vi "ini Ctrl_Str.vi"(7 "Select":enum16{"Save", "Load"}(ring), 8 "에러 입력":errorcluster caption="에러 입력(에러 없음)", 9 "값":string, 10 "키":string, 11 "섹션":string) -> (0 "에러 출력":errorcluster, 1 "값":string, 2 "경로 출력":path)   [LabVIEW 2020]
uses:
  Controls/Cmd_File path.ctl
  Controls/Cmd_File Type.ctl
  <vilib>/Utility/config.llb/Write Key (String).vi
  <vilib>/Utility/config.llb/Read Key (String).vi
  <vilib>/Utility/config.llb/NI_LVConfig.lvlib
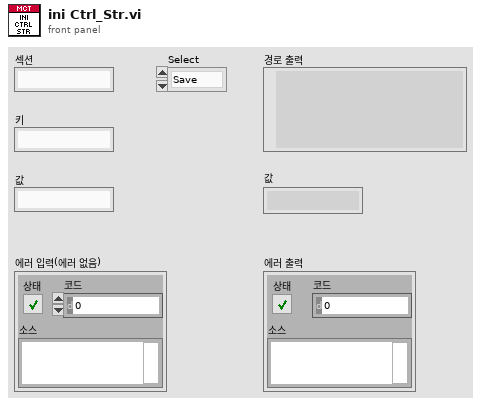
[diagram p1: front panel]
types:
  T1 = typedef "Cmd_File Type.ctl" = enum16{"엑셀", "엑셀(2003)", "텍스트", "설정", "2진", "VI", "CSV", "LOG", "폴더"}
  T2 = typedef "Cmd_File path.ctl" = enum16{"에러로그", "데이터파일경로", "성적서원본", "지난성적서", "Data Files", "경로생성", "Updater", "Template", "설정파일경로", "FTP Upload", "Update 경로", "어플리케이션"}
  T3 = typedef "NI_LVConfig.lvlib/Config Data RefNum.ctl" = refnum<k1>
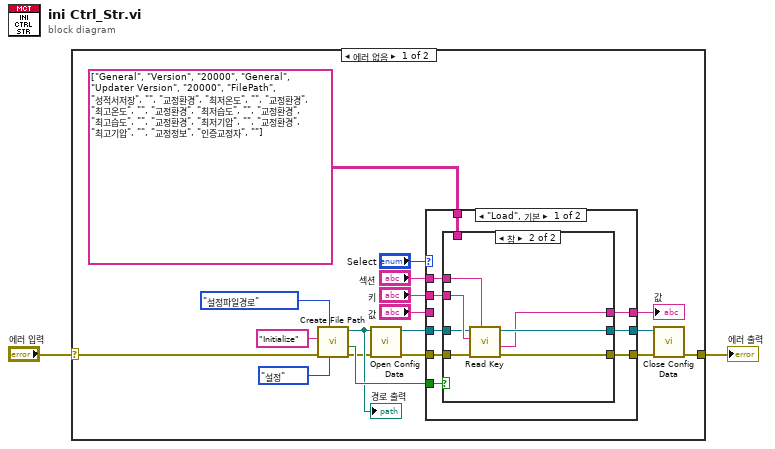
[diagram p0: block diagram]
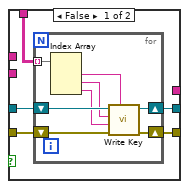
[diagram p2: hidden frame]
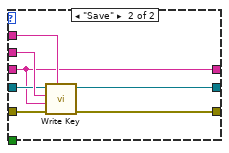
[diagram p3: hidden frame]
diagram:
  n1 = case shown="에러 없음" "에러 입력" {
    selector: "에러 입력" -> [w17 w57]
    tunnel: [w8 w57] -> w2
    frame No Error {
      n2 = call "Create File Path.vi"("파일타입"=Cmd_File_Type."설정", "항목"=Cmd_File_path."설정파일경로", "에러 입력"=w17, "문자열 in"="Initialize") -> ("error out"=w12:errorcluster, "파일존재?"=w15:bool, "파일경로"=w13:path)  [unwired: 4 in, 1 out]
      "경로 출력" <- w13
      n3 = call <vilib>:"Open Config Data.vi"("error in (no error)"=w12, "configuration file path"=w13) -> ("error out"=w10:errorcluster, "refnum"=w11:T3)  [unwired: 7 in, 1 out]
      n4 = case shown="\"Load\", 기본" "Select" {
        tunnel: [w27 w51] -> w9
        tunnel: "키" -> [w24 w56]
        tunnel: "섹션" -> [w25 w55]
        tunnel: w10 -> [w29 w54]
        tunnel: w11 -> [w28 w53]
        tunnel: w15 -> [w26 _]
        tunnel: string[][] [["General", "Version", "20000"], ["General", "Updater Version", "20000"], ["FilePath", "성적서저장", ""], ["교정환경", "최저온도", ""], ["교정환경", "최고온도", ""], ["교정환경", "최저습도", ""], ["교정환경", "최고습도", ""], ["교정환경", "최저기압", ""], ["교정환경", "최고기압", ""], ["교정정보", "인증교정자", ""]] -> [w23 _]
        tunnel: [w22 w50] -> w7
        tunnel: [w21 w52] -> w6
        tunnel: "값" -> [_ w52]
        frame "Load", Default {
          n5 = case shown="참" w26 {
            tunnel: w29 -> [w33 w46]
            tunnel: w28 -> [w32 w47]
            tunnel: [w31 w44] -> w27
            tunnel: w25 -> [_ w49]
            tunnel: w24 -> [_ w48]
            tunnel: w23 -> [w34 _]
            tunnel: [w30 w45] -> w22
            tunnel: [_ w43] -> w21
            frame False {
              n6 = for {
                shift-right: [w39] -> w31
                shift-left: w33 -> [w42]
                shift-right: [w40] -> w30
                shift-left: w32 -> [w41]
                tunnel: w34 -> [w38] mode=indexing
                n7 = Index Array(array=w38) -> (element #1=w37:string, element #2=w36:string, element #3=w35:string)  [unwired: 3 in]
                n8 = call-poly <vilib>:"Write Key.vi"("section"=w37, "error in (no error)"=w42, "value"=w35, "key"=w36, "refnum"=w41) -> ("error out"=w39:errorcluster, "refnum out"=w40:T3)  [unwired: 4 in, 1 out]
              }
            }
            frame True {
              n9 = call-poly <vilib>:"Read Key.vi"("section"=w49, "error in (no error)"=w46, "key"=w48, "refnum"=w47) -> ("error out"=w44:errorcluster, "value"=w43:string, "refnum out"=w45:T3)  [unwired: 4 in, 1 out]
            }
          }
        }
        frame "Save" {
          n10 = call-poly <vilib>:"Write Key.vi"("section"=w55, "error in (no error)"=w54, "value"=w52, "key"=w56, "refnum"=w53) -> ("error out"=w51:errorcluster, "refnum out"=w50:T3)  [unwired: 4 in, 1 out]
        }
      }
      "값" <- w6
      n11 = call <vilib>:"Close Config Data.vi"("error in (no error)"=w9, "refnum"=w7) -> ("error out"=w8:errorcluster)  [unwired: 8 in, 1 out]
    }
    frame Error {
    }
  }
  "에러 출력" <- w2
